vi "USB_CAN_ABOUT_DLG.vi"(11 "Verinfo":string) -> ()   [LabVIEW 2011]
doc: "ID=0x6002"
uses:
  XSuperLink/xcontrol/XSuperLink.xctl
panel:
  out "label1":string="版权所有（C）2017-2019，珠海创芯科技有限公司"
  out "label2":string="USB-CAN Tool V2.01"
  out "e-mail":string(xcontrol) caption="技术支持邮箱："
  in  "OK":bool
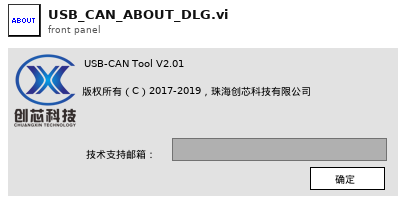
[diagram p1: front panel]
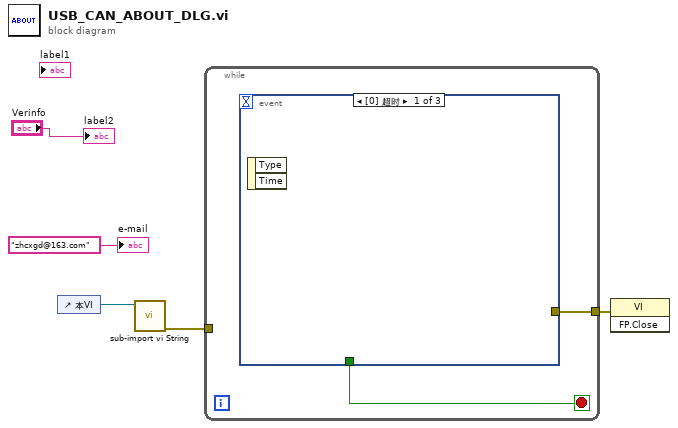
[diagram p0: block diagram]
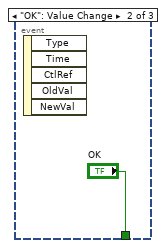
[diagram p2: hidden frame]
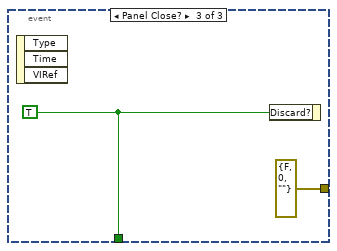
[diagram p3: hidden frame]
diagram:
  n1 = control-ref of="本VI"() -> (w3:refnum<vi>)
  n2 = call "sub-import vi String.vi"("vi ref"=w3) -> ("error out"=w2:errorcluster)  [unwired: 10 in]
  n3 = while {
    tunnel: [w6] -> w5
    tunnel: w2 -> [_]
    stop <- w7 stop-if-true
    n4 = event shown="[0] 超时" {
      selector: _ -> [_ _ _]
      dyn-events: _ -> [_ _ _]
      timeout: _ -> [_ _ _]
      tunnel: [_ "OK" w10] -> w7
      tunnel: [_ _ errorcluster {"status"=FALSE, "code"=0, "source"=""} ("错误输入（无错误）")] -> w6
      event Timeout {
        n5 = event-data() -> ()  [unwired: 1 in, 2 out]
      }
      event "OK": Value Change {
        n6 = event-data() -> ()  [unwired: 1 in, 5 out]
      }
      event Panel Close? {
        w10 = TRUE ("放弃？")
        n7 = event-data() -> ()  [unwired: 1 in, 3 out]
        n8 = event-data("Discard?"=w10) -> ()  [unwired: 1 in, 1 out]
      }
    }
  }
  n9 = invoke class="VI" method="FP.Close"(error in=w5) -> ()  [unwired: 2 in, 3 out]
  "e-mail" <- "zhcxgd@163.com" ("淘宝店铺：")
  "label2" <- "Verinfo"
